vi "Read Runtime Data.vi"(7 "Section Name":string="PluginSpecific", 8 "error in":errorcluster, 10 "Curr Cal Type":i32=-1, 11 "Config File Data In":T1(array[cluster])) -> (0 "error out":errorcluster, 2 "Runtime Data Out":T2, 3 "Config Data Out":T1(array[cluster]))   [LabVIEW 2020, in "GUCalibration2.lvlib"]
uses:
  GUCalibration2.lvlib
  Controls/Config Data Type.ctl
  Utilities/Read Key String.vi
  Utilities/Read Key Boolean.vi
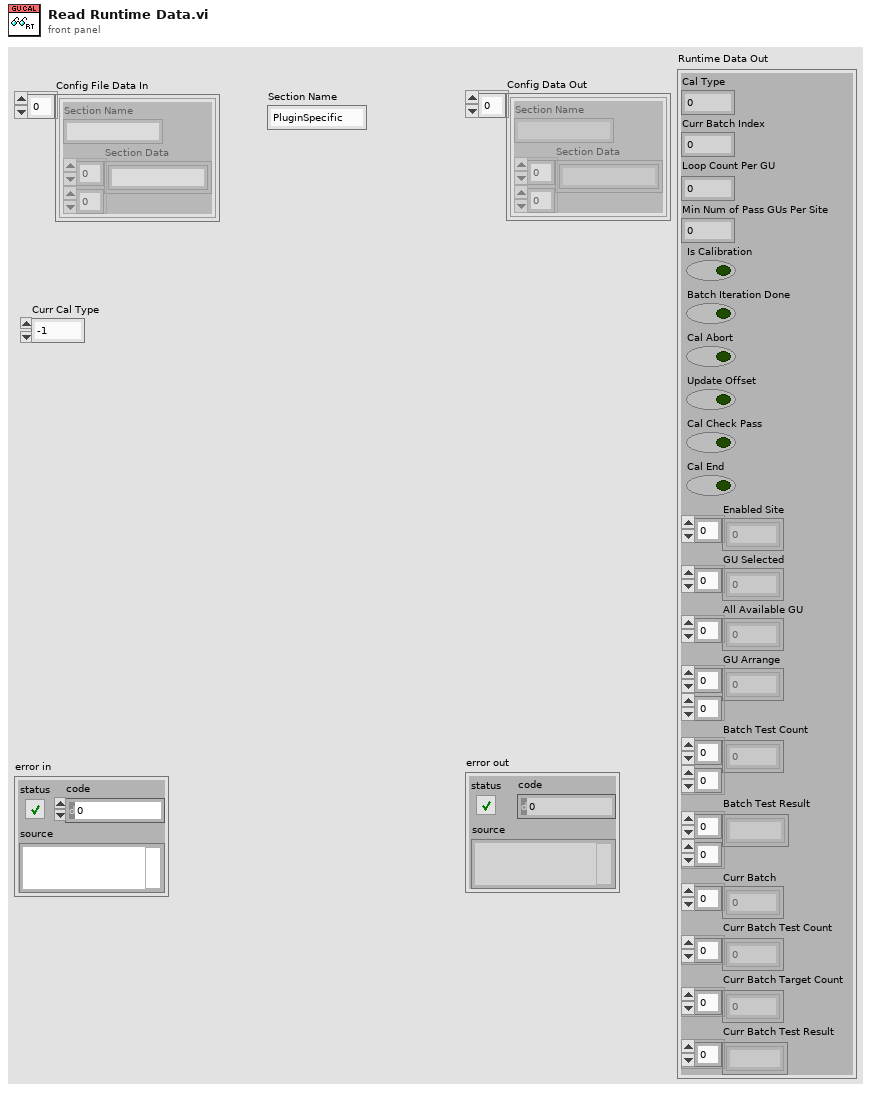
[diagram p1: front panel]
types:
  T1 = cluster{"Section Name":string, "Section Data":string[][]}[]
  T2 = typedef "GUCalibration2.lvlib/Config Data Type.ctl" = cluster{"Cal Type":i32, "Curr Batch Index":i32, "Loop Count Per GU":i32, "Min Num of Pass GUs Per Site":i32, "Is Calibration":bool, "Batch Iteration Done":bool, "Cal Abort":bool, "Update Offset":bool, "Cal Check Pass":bool, "Cal End":bool, "Enabled Site":i32[], "GU Selected":i32[], "All Available GU":i32[], "GU Arrange":i32[][], "Batch Test Count":i32[][], "Batch Test Result":string[][], "Curr Batch":i32[], "Curr Batch Test Count":i32[], "Curr Batch Target Count":i32[], "Curr Batch Test Result":string[]}
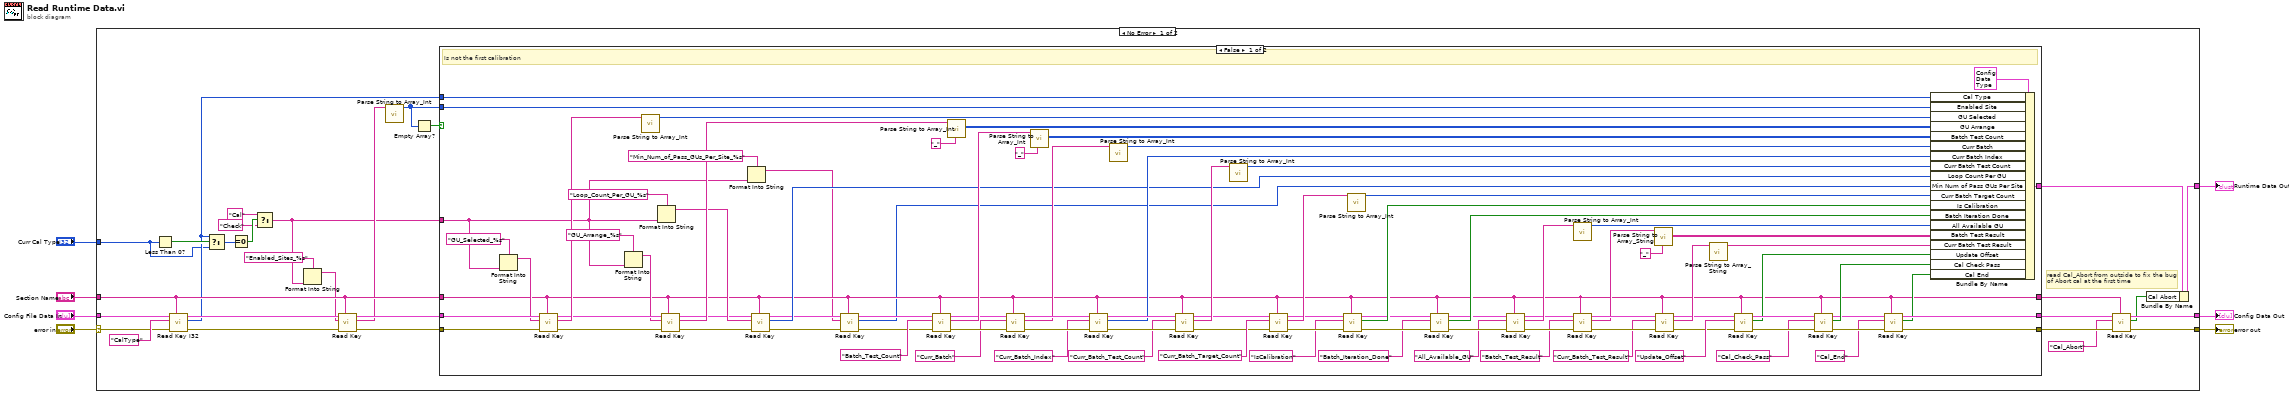
[diagram p0: block diagram]
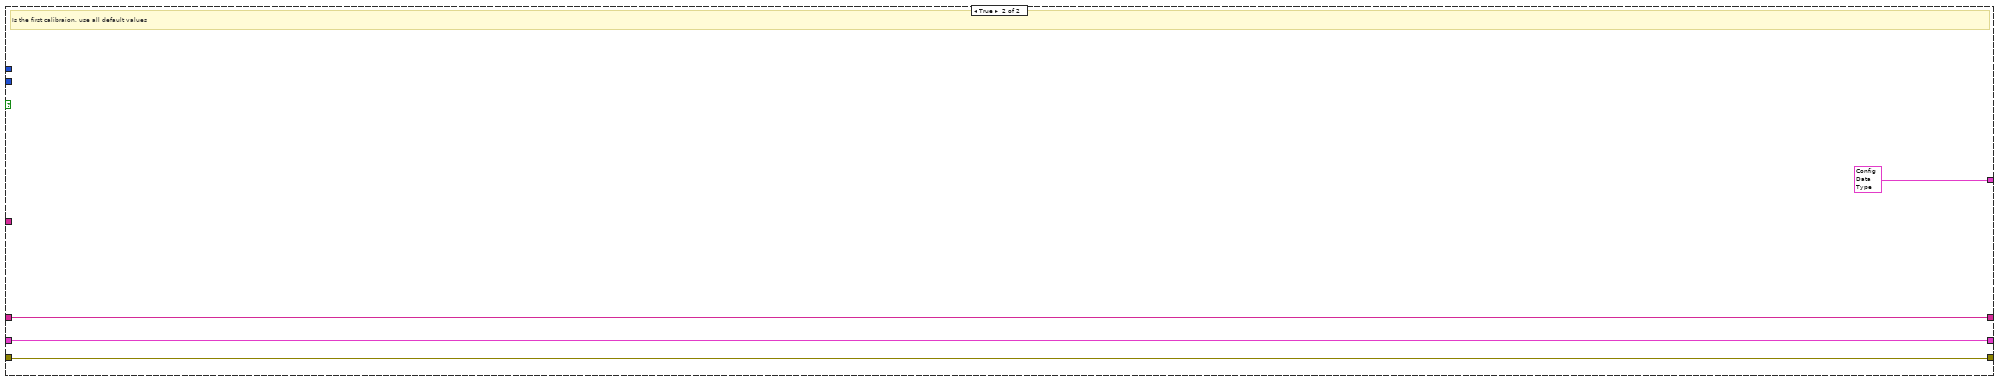
[diagram p2: hidden frame]
diagram:
  n1 = case shown="No Error" "error in" {
    selector: "error in" -> [w34 w135]
    tunnel: "Config File Data In" -> [w36 w134]
    tunnel: "Section Name" -> [w29 _]
    tunnel: [w18 w135] -> w5
    tunnel: [w14 _] -> w4
    tunnel: [w17 w134] -> w2
    tunnel: "Curr Cal Type" -> [w23 _]
    frame No Error {
      # "read Cal_Abort from outside to fix the bug\nof Abort cal at the first time"
      n2 = Less Than 0?(x=w23) -> (x < 0?=w25:bool)
      n3 = call "Read Key I32.vi"("Section Name"=w29, "error in (no error)"=w34, "Key Names"="CalType" ("Section Name"), "Config Data"=w36) -> ("error out"=w32:errorcluster, "Key Value out"=w24:i32, "Config Data dup"=w33:T1)  [unwired: 3 in, 2 out]
      n4 = Select(t=w24, s=w25, f=w23) -> (s? t:f=w12:i32)
      n5 = Equal To 0?(x=w12) -> (x = 0?=w11:bool)
      n6 = Select(t="Cal" ("Section Name"), s=w11, f="Check" ("Section Name")) -> (s? t:f=w8:string)
      n7 = Format Into String(format string="Enabled_Sites_%s" ("Section Name"), w8) -> (resulting string=w21:string)  [unwired: 2 in, 1 out]
      n8 = call-poly "Read Key.vi"("Section Name"=w29, "error in (no error)"=w32, "Key Names"=w21, "Config Data"=w33) -> ("error out"=w30:errorcluster, "Key Val out"=w28:string, "Config Data dup"=w31:T1)  [unwired: 3 in, 2 out]
      n9 = call "Parse String to Array_Int.vi"("String Input"=w28) -> ("Data 1"=w27:i32[])  [unwired: 9 in, 1 out]
      n10 = Empty Array?(array=w27) -> (empty?=w26:bool)
      n11 = case shown="False" w26 {
        tunnel: w31 -> [w129 w133]
        tunnel: w30 -> [w128 w132]
        tunnel: [w107 T2 {"Cal Type"=0, "Curr Batch Index"=0, "Loop Count Per GU"=1, "Min Num of Pass GUs Per Site"=0, "Is Calibration"=FALSE, "Batch Iteration Done"=FALSE, "Cal Abort"=FALSE, "Update Offset"=FALSE, "Cal Check Pass"=FALSE, "Cal End"=FALSE, "Enabled Site"=[], "GU Selected"=[], "All Available GU"=[], "GU Arrange"=[], "Batch Test Count"=[], "Batch Test Result"=[], "Curr Batch"=[], "Curr Batch Test Count"=[], "Curr Batch Target Count"=[], "Curr Batch Test Result"=[]} ("Cluster")] -> w35
        tunnel: w24 -> [w106 _]
        tunnel: w29 -> [w42 w130]
        tunnel: [w61 w133] -> w16
        tunnel: [w62 w132] -> w19
        tunnel: w27 -> [w91 _]
        tunnel: w8 -> [w40 _]
        tunnel: [w42 w130] -> w20
        frame False {
          # "Is not the first calibration"
          n12 = Format Into String(format string="GU_Selected_%s" ("Section Name"), w40) -> (resulting string=w57:string)  [unwired: 2 in, 1 out]
          n13 = call-poly "Read Key.vi"("Section Name"=w42, "error in (no error)"=w128, "Key Names"=w57, "Config Data"=w129) -> ("error out"=w125:errorcluster, "Key Val out"=w127:string, "Config Data dup"=w126:T1)  [unwired: 3 in, 2 out]
          n14 = Format Into String(format string="GU_Arrange_%s" ("Section Name"), w40) -> (resulting string=w55:string)  [unwired: 2 in, 1 out]
          n15 = call "Parse String to Array_Int.vi"("String Input"=w127) -> ("Data 1"=w105:i32[])  [unwired: 9 in, 1 out]
          n16 = Format Into String(format string="Loop_Count_Per_GU_%s" ("Section Name"), w40) -> (resulting string=w53:string)  [unwired: 2 in, 1 out]
          n17 = call-poly "Read Key.vi"("Section Name"=w42, "error in (no error)"=w125, "Key Names"=w55, "Config Data"=w126) -> ("error out"=w50:errorcluster, "Key Val out"=w124:string, "Config Data dup"=w49:T1)  [unwired: 3 in, 2 out]
          n18 = Format Into String(format string="Min_Num_of_Pass_GUs_Per_Site_%s" ("Section Name"), w40) -> (resulting string=w39:string)  [unwired: 2 in, 1 out]
          n19 = call-poly "Read Key.vi"("Section Name"=w42, "error in (no error)"=w50, "Key Names"=w53, "Config Data"=w49) -> ("error out"=w46:errorcluster, "Key Value out"=w99:i32, "Config Data dup"=w44:T1)  [unwired: 3 in, 2 out]
          n20 = call-poly "Read Key.vi"("Section Name"=w42, "error in (no error)"=w46, "Key Names"=w39, "Config Data"=w44) -> ("error out"=w45:errorcluster, "Key Value out"=w38:i32, "Config Data dup"=w43:T1)  [unwired: 3 in, 2 out]
          n21 = call-poly "Read Key.vi"("Section Name"=w42, "error in (no error)"=w45, "Key Names"="Batch_Test_Count" ("Section Name"), "Config Data"=w43) -> ("error out"=w120:errorcluster, "Key Val out"=w122:string, "Config Data dup"=w121:T1)  [unwired: 3 in, 2 out]
          n22 = call "Parse String to Array_Int.vi"("Spliter 2"="_", "String Input"=w124) -> ("Data 2"=w104:i32[][])  [unwired: 8 in, 1 out]
          n23 = call-poly "Read Key.vi"("Section Name"=w42, "error in (no error)"=w120, "Key Names"="Curr_Batch" ("Section Name"), "Config Data"=w121) -> ("error out"=w117:errorcluster, "Key Val out"=w116:string, "Config Data dup"=w118:T1)  [unwired: 3 in, 2 out]
          n24 = call "Parse String to Array_Int.vi"("Spliter 2"="_", "String Input"=w122) -> ("Data 2"=w103:i32[][])  [unwired: 8 in, 1 out]
          n25 = call-poly "Read Key.vi"("Section Name"=w42, "error in (no error)"=w117, "Key Names"="Curr_Batch_Index" ("Section Name"), "Config Data"=w118) -> ("error out"=w113:errorcluster, "Key Value out"=w101:i32, "Config Data dup"=w114:T1)  [unwired: 3 in, 2 out]
          n26 = call "Parse String to Array_Int.vi"("String Input"=w116) -> ("Data 1"=w102:i32[])  [unwired: 9 in, 1 out]
          n27 = call-poly "Read Key.vi"("Section Name"=w42, "error in (no error)"=w113, "Key Names"="Curr_Batch_Test_Count" ("Section Name"), "Config Data"=w114) -> ("error out"=w48:errorcluster, "Key Val out"=w111:string, "Config Data dup"=w47:T1)  [unwired: 3 in, 2 out]
          n28 = call "Parse String to Array_Int.vi"("String Input"=w111) -> ("Data 1"=w100:i32[])  [unwired: 9 in, 1 out]
          n29 = call-poly "Read Key.vi"("Section Name"=w42, "error in (no error)"=w48, "Key Names"="Curr_Batch_Target_Count" ("Section Name"), "Config Data"=w47) -> ("error out"=w94:errorcluster, "Key Val out"=w97:string, "Config Data dup"=w95:T1)  [unwired: 3 in, 2 out]
          n30 = call-poly "Read Key.vi"("Section Name"=w42, "error in (no error)"=w94, "Key Names"="IsCalibration" ("Section Name"), "Config Data"=w95) -> ("error out"=w89:errorcluster, "Key Value out"=w92:bool, "Config Data dup"=w90:T1)  [unwired: 3 in, 2 out]
          n31 = call "Parse String to Array_Int.vi"("String Input"=w97) -> ("Data 1"=w96:i32[])  [unwired: 9 in, 1 out]
          n32 = call-poly "Read Key.vi"("Section Name"=w42, "error in (no error)"=w89, "Key Names"="Batch_Iteration_Done" ("Section Name"), "Config Data"=w90) -> ("error out"=w85:errorcluster, "Key Value out"=w87:bool, "Config Data dup"=w86:T1)  [unwired: 3 in, 2 out]
          n33 = call-poly "Read Key.vi"("Section Name"=w42, "error in (no error)"=w85, "Key Names"="All_Available_GU" ("Section Name"), "Config Data"=w86) -> ("error out"=w80:errorcluster, "Key Val out"=w83:string, "Config Data dup"=w81:T1)  [unwired: 3 in, 2 out]
          n34 = call "Parse String to Array_Int.vi"("String Input"=w83) -> ("Data 1"=w82:i32[])  [unwired: 9 in, 1 out]
          n35 = call-poly "Read Key.vi"("Section Name"=w42, "error in (no error)"=w80, "Key Names"="Batch_Test_Result" ("Section Name"), "Config Data"=w81) -> ("error out"=w78:errorcluster, "Key Val out"=w75:string, "Config Data dup"=w79:T1)  [unwired: 3 in, 2 out]
          n36 = call "Parse String to Array_String.vi"("Spliter 2"="_", "String Input"=w75) -> ("Data 2"=w74:string[][])  [unwired: 8 in, 1 out]
          n37 = call-poly "Read Key.vi"("Section Name"=w42, "error in (no error)"=w78, "Key Names"="Curr_Batch_Test_Result" ("Section Name"), "Config Data"=w79) -> ("error out"=w51:errorcluster, "Key Val out"=w71:string, "Config Data dup"=w52:T1)  [unwired: 3 in, 2 out]
          n38 = call "Parse String to Array_String.vi"("String Input"=w71) -> ("Data 1"=w72:string[])  [unwired: 9 in, 1 out]
          n39 = call-poly "Read Key.vi"("Section Name"=w42, "error in (no error)"=w51, "Key Names"="Update_Offset" ("Section Name"), "Config Data"=w52) -> ("error out"=w69:errorcluster, "Key Value out"=w67:bool, "Config Data dup"=w70:T1)  [unwired: 3 in, 2 out]
          n40 = call-poly "Read Key.vi"("Section Name"=w42, "error in (no error)"=w69, "Key Names"="Cal_Check_Pass" ("Section Name"), "Config Data"=w70) -> ("error out"=w63:errorcluster, "Key Value out"=w65:bool, "Config Data dup"=w64:T1)  [unwired: 3 in, 2 out]
          n41 = call-poly "Read Key.vi"("Section Name"=w42, "error in (no error)"=w63, "Key Names"="Cal_End" ("Section Name"), "Config Data"=w64) -> ("error out"=w62:errorcluster, "Key Value out"=w59:bool, "Config Data dup"=w61:T1)  [unwired: 3 in, 2 out]
          n42 = Bundle By Name(cluster=T2 {"Cal Type"=0, "Curr Batch Index"=0, "Loop Count Per GU"=0, "Min Num of Pass GUs Per Site"=0, "Is Calibration"=FALSE, "Batch Iteration Done"=FALSE, "Cal Abort"=FALSE, "Update Offset"=FALSE, "Cal Check Pass"=FALSE, "Cal End"=FALSE, "Enabled Site"=[], "GU Selected"=[], "All Available GU"=[], "GU Arrange"=[], "Batch Test Count"=[], "Batch Test Result"=[], "Curr Batch"=[], "Curr Batch Test Count"=[], "Curr Batch Target Count"=[], "Curr Batch Test Result"=[]} ("Cluster"), "Cal Type"=w106, "Enabled Site"=w91, "GU Selected"=w105, "GU Arrange"=w104, "Batch Test Count"=w103, "Curr Batch"=w102, "Curr Batch Index"=w101, "Curr Batch Test Count"=w100, "Loop Count Per GU"=w99, "Min Num of Pass GUs Per Site"=w38, "Curr Batch Target Count"=w96, "Is Calibration"=w92, "Batch Iteration Done"=w87, "All Available GU"=w82, "Batch Test Result"=w74, "Curr Batch Test Result"=w72, "Update Offset"=w67, "Cal Check Pass"=w65, "Cal End"=w59) -> (w107:T2)
        }
        frame True {
          # "Is the first calibraion, use all default values"
        }
      }
      n43 = call-poly "Read Key.vi"("Section Name"=w20, "error in (no error)"=w19, "Key Names"="Cal_Abort" ("Section Name"), "Config Data"=w16) -> ("error out"=w18:errorcluster, "Key Value out"=w13:bool, "Config Data dup"=w17:T1)  [unwired: 3 in, 2 out]
      n44 = Bundle By Name(cluster=w35, "Cal Abort"=w13) -> (w14:T2)
    }
    frame Error {
    }
  }
  "error out" <- w5
  "Runtime Data Out" <- w4
  "Config Data Out" <- w2
